vi "Read Additional Send Headers.vi"(8 "error in (no error)":errorcluster, 11 "Websocket Handler in":refnum<class "Websocket Handler.lvclass">) -> (0 "error out":errorcluster, 2 "Additional Send Headers":T1[](array[typedef]), 3 "Websocket Handler out":refnum<class "Websocket Handler.lvclass">)   [LabVIEW 2020, in "wamplv.lvlib" / "Websocket Handler.lvclass"]
uses:
  Websocket Handler.lvclass
  <vilib>/MediaMongrels Ltd/WebSockets/WebSockets/WebSocket/Headers.ctl
  <vilib>/MediaMongrels Ltd/WebSockets/WebSockets/WebSocket/WebSocket.lvclass
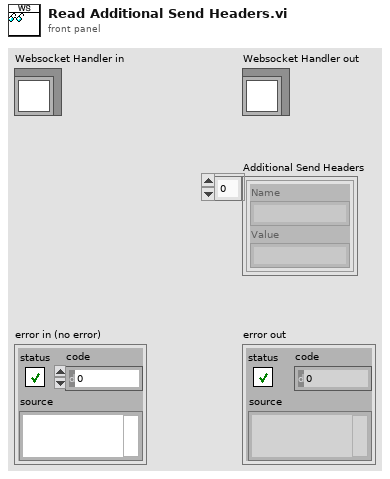
[diagram p1: front panel]
types:
  T1 = typedef "WebSockets.lvlib/WebSocket.lvclass/Headers.ctl" = cluster{"Name":string, "Value":string}
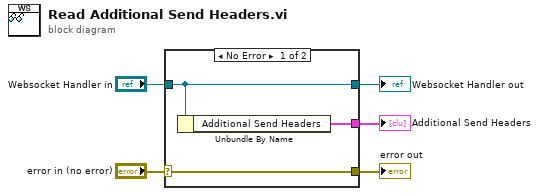
[diagram p0: block diagram]
diagram:
  n1 = case shown="No Error" "error in (no error)" {
    selector: "error in (no error)" -> [w8 w9]
    tunnel: [w8 w9] -> w4
    tunnel: [w7 w10] -> w2
    tunnel: "Websocket Handler in" -> [w7 w10]
    tunnel: [w6 _] -> w1
    frame No Error {
      n2 = Unbundle By Name(w7) -> ("Additional Send Headers"=w6:T1[])
    }
    frame Error {
    }
  }
  "error out" <- w4
  "Websocket Handler out" <- w2
  "Additional Send Headers" <- w1
